vi "Draw Tangent Line.vi"(10 "Cluster":cluster{dbl, dbl}, 11 "Numeric":dbl) -> (3 "Array":cluster{dbl, dbl}[](array[cluster]))   [LabVIEW 2018]
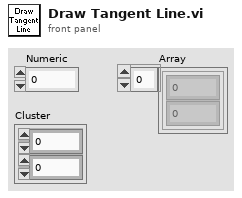
[diagram p1: front panel]
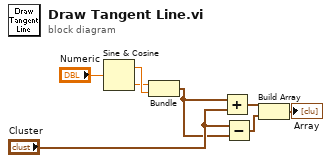
[diagram p0: block diagram]
diagram:
  n1 = Sine & Cosine(0:"Numeric") -> (1:w2:dbl, 2:w1:dbl)
  n2 = Bundle(w1, w2) -> (w7:cluster{dbl, dbl})  [unwired: 1 in]
  n3 = Add(x=w7, y="Cluster") -> (x+y=w3:cluster{dbl, dbl})
  n4 = Subtract(x="Cluster", y=w7) -> (x-y=w4:cluster{dbl, dbl})
  n5 = Build Array(w3, w4) -> (→"Array":cluster{dbl, dbl}[])
